vi "Create Errors.vi"(1 "Include call chain?":bool, 2 "Error Message Type":T1, 3 "Number of different error codes":u32) -> (0 "Errors":errorcluster[](array[cluster]))   [LabVIEW 2023, in "Error Manager.lvlib" / "Anti-Spam Tester (AST).lvlib"]
doc: "Blank VI with error handling."
uses:
  Anti-Spam Tester (AST).lvlib
  Spam Error Message Type (enum).ctl
panel:
  # "Input\nInputs to the VI"
  # "Development\nControls or indicators that are useful for development or testing, but which are not outputs of the VI."
  # "Output\nOutputs of the VI"
  # "Description\n\nBlank VI with error handling case. \n\nSummarize the use of this VI in this space."
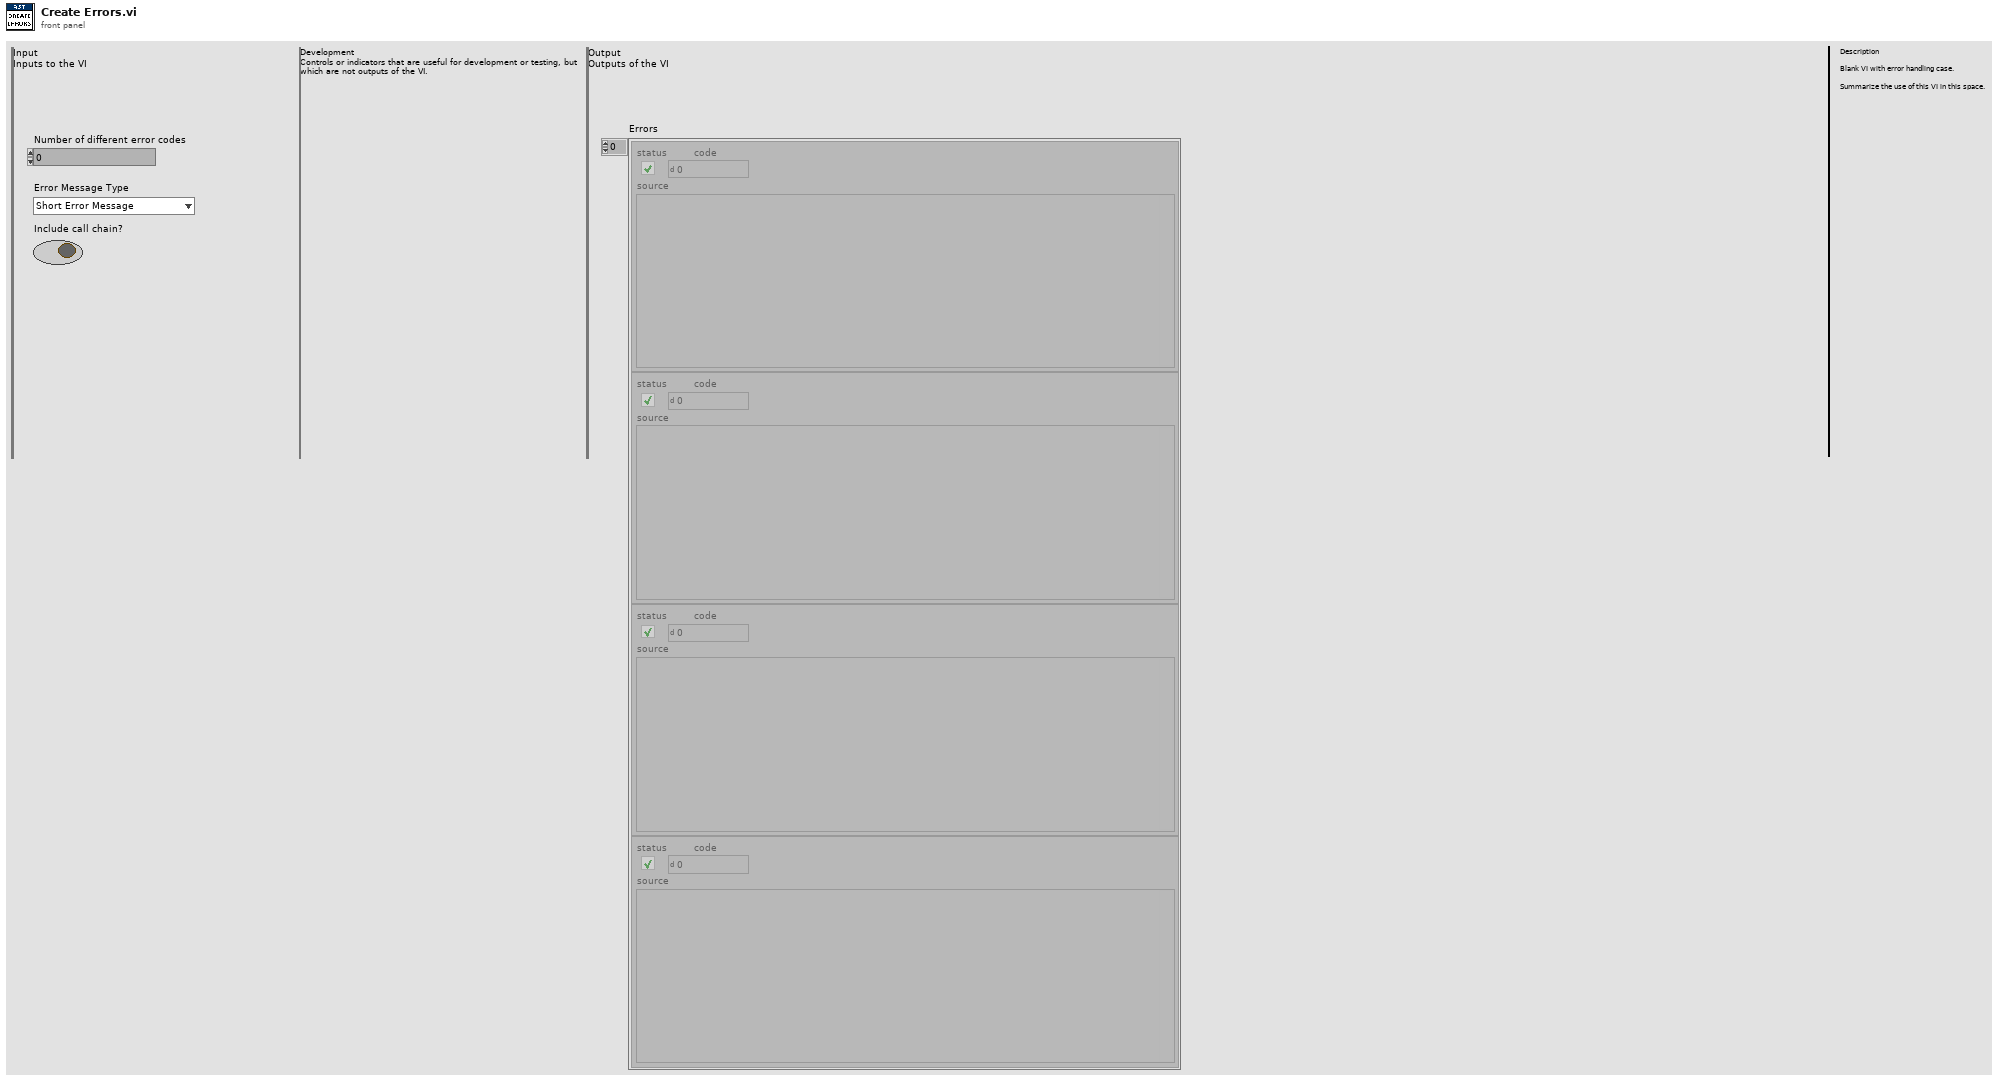
[diagram p1: front panel]
types:
  T1 = typedef "Error Manager.lvlib/Anti-Spam Tester (AST).lvlib/Spam Error Message Type (enum).ctl" = enum16{"Short Error Message", "Long Error Message"}
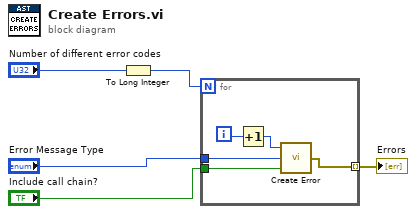
[diagram p0: block diagram]
diagram:
  n1 = To Long Integer(number="Number of different error codes") -> (32bit integer=w4:i32)
  n2 = for {
    N: w4 -> [_]
    tunnel: "Error Message Type" -> [w8]
    tunnel: "Include call chain?" -> [w7]
    tunnel: [w6] -> w1 mode=indexing
    i -> [w10]
    n3 = Increment(x=w10) -> (x+1=w9:i32)
    n4 = call "Create Error.vi"("Include call chain?"=w7, "Error Message Type"=w8, "Error iteration number (i)"=w9) -> ("Error"=w6:errorcluster)
  }
  "Errors" <- w1
